vi "getCurrentPositionOfDangerEnemies.vi"(7 "Robot":refnum<class "Robot.lvclass">, 8 "error in (no error)":errorcluster, 9 "RobotRef":refnum<class "Robot.lvclass">[](array[class]), 10 "dangerEnemies":T1[](array[typedef]), 11 "MarkerSkill in":refnum<class "MarkerSkill.lvclass">) -> (0 "error out":errorcluster, 2 "positionToMark":dbl[](array[numeric]), 3 "MarkerSkill out":refnum<class "MarkerSkill.lvclass">)   [LabVIEW 2021, in "MarkerSkill.lvclass"]
uses:
  MarkerSkill.lvclass
  dangerEnemy.ctl
  Robot_class/Robot.lvclass
  D:/RoboIme/horie/SSL_AI/Object_class/Object.lvclass
  Robot_class/Robot.lvclass/Robot.ctl
  Object_class/Object.lvclass/Object.ctl
  Robot_class/Read id.vi
  Object_class/Read position(x,y).vi
  Utilities_class/Utilities.lvclass
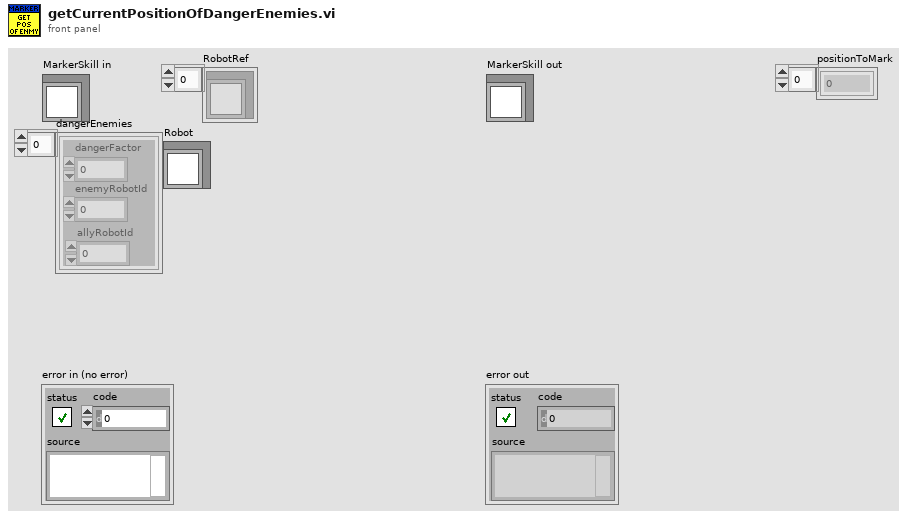
[diagram p1: front panel]
types:
  T1 = typedef "dangerEnemy.ctl" = cluster{"dangerFactor":dbl, "allyRobotId":i32, "enemyRobotId":i32}
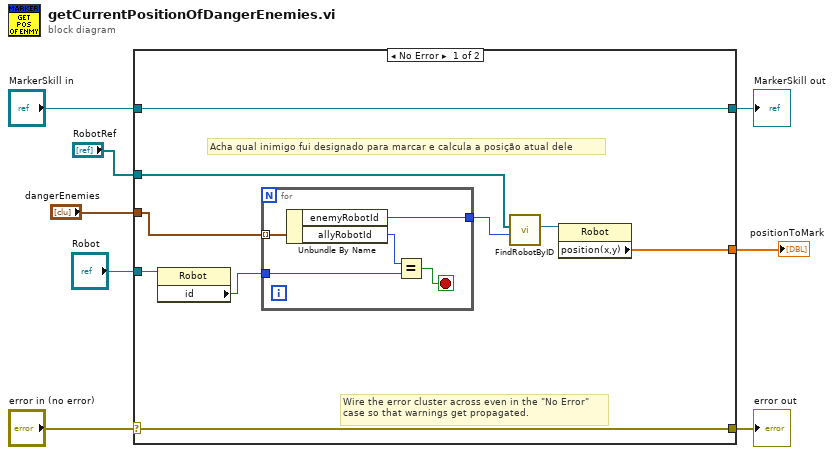
[diagram p0: block diagram]
diagram:
  n1 = case shown="No Error" "error in (no error)" {
    selector: "error in (no error)" -> [w16 w24]
    tunnel: [w16 w24] -> w7
    tunnel: [w17 w23] -> w5
    tunnel: "MarkerSkill in" -> [w17 w23]
    tunnel: "dangerEnemies" -> [w12 _]
    tunnel: [w15 _] -> w1
    tunnel: "RobotRef" -> [w14 _]
    tunnel: "Robot" -> [w11 _]
    frame No Error {
      # "Acha qual inimigo fui designado para marcar e calcula a posição atual dele"
      # "Wire the error cluster across even in the \"No Error\"\ncase so that warnings get propagated."
      n2 = property class="Robot"(reference=w11) -> ("id"=w10:i32)  [unwired: 1 in, 2 out]
      n3 = for {
        tunnel: w12 -> [w22] mode=indexing
        tunnel: w10 -> [w20]
        tunnel: [w18] -> w9
        stop <- w19 stop-if-true
        n4 = Unbundle By Name(w22) -> ("enemyRobotId"=w18:i32, "allyRobotId"=w21:i32)
        n5 = Equal?(x=w21, y=w20) -> (x = y?=w19:bool)
      }
      n6 = call "FindRobotByID.vi"("id"=w9, "RobotRef"=w14) -> ("Robot"=w13:refnum<class "Robot.lvclass">)  [unwired: 6 in, 3 out]
      n7 = property class="Robot"(reference=w13) -> ("position(x,y)"=w15:dbl[])  [unwired: 1 in, 2 out]
    }
    frame Error {
    }
  }
  "error out" <- w7
  "MarkerSkill out" <- w5
  "positionToMark" <- w1
